vi "SQLite List Template.vi"(6 "Range":T1, 7 "Filter":cluster{}, 8 "Error in":errorcluster, 10 "Fields":string[](array[combo]), 11 "SQLite Connection in":refnum<class "Connection.lvclass">) -> (0 "Error out":errorcluster, 2 "Data out":variant[][](array[variant]), 3 "SQLite Connection out":refnum<class "Connection.lvclass">)   [LabVIEW 2021]
uses:
  <vilib>/drjdpowell/SQLite Library/SQL Statement/SQL Statement.lvclass
  <vilib>/drjdpowell/SQLite Library/SQL Connection/Connection.lvclass
  edt.lib/sqlite.lib/EDT SQLite+.lvlib
  edt.lib/sqlite.lib/SQLite Range.ctl
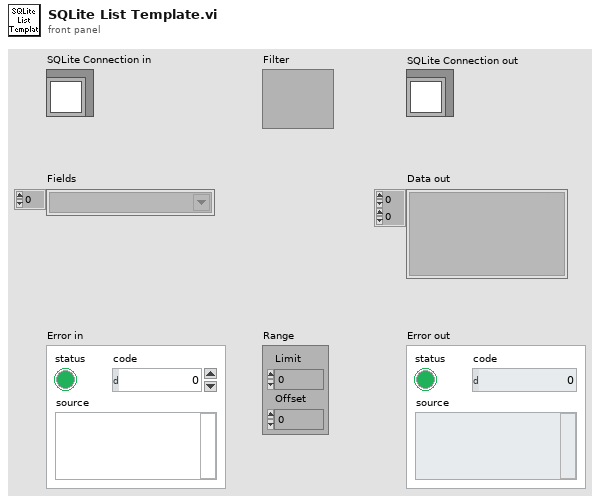
[diagram p1: front panel]
types:
  T1 = typedef "EDT SQLite+.lvlib/SQLite Range.ctl" = cluster{"Limit":i32, "Offset":i32}
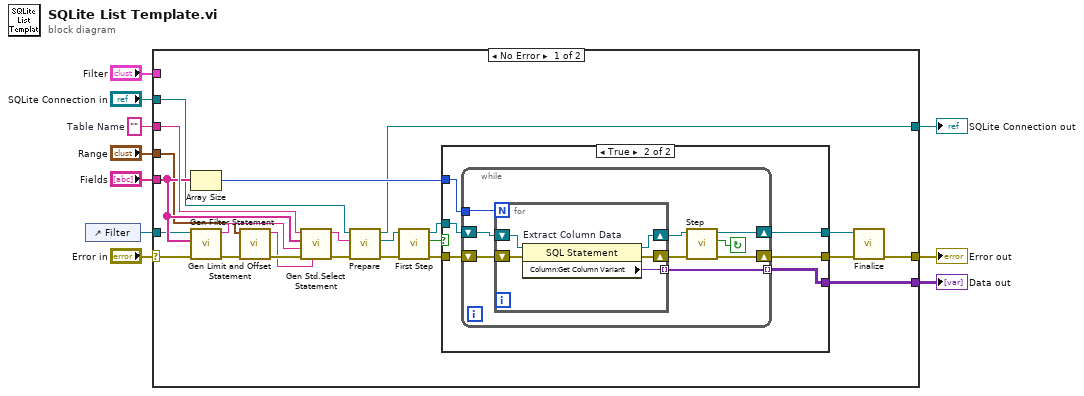
[diagram p0: block diagram]
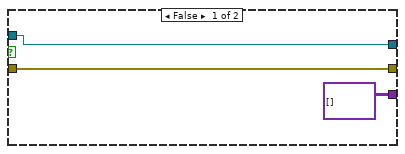
[diagram p2: hidden frame]
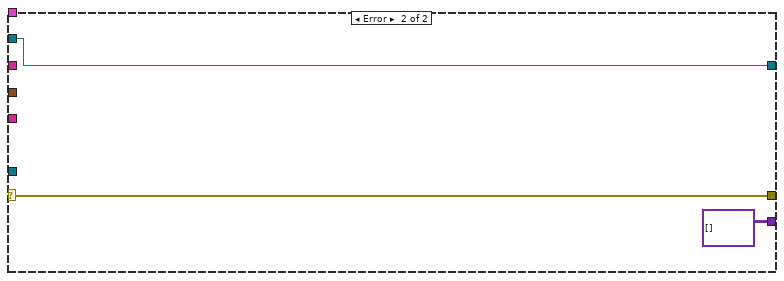
[diagram p3: hidden frame]
diagram:
  w5 = ""  # Table Name
  n1 = control-ref of="Filter"() -> (w4:refnum<vi>)
  n2 = case shown="No Error" "Error in" {
    selector: "Error in" -> [w20 w59]
    tunnel: [w26 w59] -> w9
    tunnel: "Filter" -> [_ _]
    tunnel: [w25 variant[][] []] -> w2
    tunnel: "SQLite Connection in" -> [w17 w58]
    tunnel: [w16 w58] -> w6
    tunnel: w5 -> [w23 _]
    tunnel: w4 -> [w21 _]
    tunnel: "Fields" -> [w22 _]
    tunnel: "Range" -> [w13 _]
    frame No Error {
      n3 = Array Size(array=w22) -> (size(s)=w18:i32)
      n4 = call "Gen Filter Statement.vi"("error in"=w20, "Columns"=w22, "Filter Cluster in"=w21) -> ("error out"=w15:errorcluster, "Filter String"=w19:string)  [unwired: 7 in]
      n5 = call "Gen Limit and Offset Statement.vi"("error in"=w15, "Range"=w13) -> ("error out"=w14:errorcluster, "Limit and Offset Statement"=w12:string)  [unwired: 8 in]
      n6 = call "Gen Std.Select Statement.vi"("Range String"=w12, "Error in"=w14, "Filter String"=w19, "Fields"=w22, "Table Name"=w23) -> ("Error out"=w11:errorcluster, "String"=w24:string)  [unwired: 5 in]
      n7 = call <vilib>:"Prepare.vi"("error in (no error)"=w11, "SQL"=w24, "SQLite Connection in"=w17) -> ("error out"=w31:errorcluster, "SQL Statement"=w30:refnum<class "SQL Statement.lvclass">, "SQLite Connection"=w16:refnum<class "Connection.lvclass">)  [unwired: 4 in, 2 out]
      n8 = call <vilib>:"First Step.vi"("error in (no error)"=w31, "SQL Statement in"=w30) -> ("error out"=w28:errorcluster, "Row returned"=w27:bool, "SQL Statement"=w29:refnum<class "SQL Statement.lvclass">)  [unwired: 7 in]
      n9 = case "Results returned?" shown="True" w27 {
        tunnel: [w36 w42] -> w32
        tunnel: [w35 w41] -> w33
        tunnel: w29 -> [w36 w40]
        tunnel: w28 -> [w35 w39]
        tunnel: [variant[][] [] w38] -> w25
        tunnel: w18 -> [_ w37]
        frame False {
        }
        frame True {
          n10 = while {
            tunnel: [w46] -> w38 mode=indexing
            shift-right: [w51] -> w42
            shift-left: w40 -> [w49]
            shift-right: [w50] -> w41
            shift-left: w39 -> [w48]
            tunnel: w37 -> [w43]
            stop <- w44 continue-if-true
            n11 = for {
              N: w43 -> [_]
              shift-right: [w56] -> w47
              shift-left: w49 -> [w55]
              shift-right: [w53] -> w45
              shift-left: w48 -> [w54]
              tunnel: [w52] -> w46 mode=indexing
              n12 = property on="Extract Column Data" class="SQL Statement"(reference=w55, error in=w54) -> (reference out=w56:refnum<class "SQL Statement.lvclass">, error out=w53:errorcluster, "Column:Get Column Variant"=w52:variant)
            }
            n13 = call <vilib>:"Step.vi"("error in (no error)"=w45, "SQL Statement in"=w47) -> ("error out"=w50:errorcluster, "Row returned"=w44:bool, "SQL Statement"=w51:refnum<class "SQL Statement.lvclass">)  [unwired: 7 in]
          }
        }
      }
      n14 = call <vilib>:"Finalize.vi"("error in (no error)"=w33, "SQL Statement in"=w32) -> ("error out"=w26:errorcluster)  [unwired: 9 in]
    }
    frame Error {
    }
  }
  "Error out" <- w9
  "SQLite Connection out" <- w6
  "Data out" <- w2
